vi "Pigeon2Configurator.vi"(6 "timeoutSeconds":dbl=0.05, 8 "error in":errorcluster, 10 "DeviceConfiguration":T2, 11 "DeviceReference":T1) -> (0 "error out":errorcluster)   [LabVIEW 2023]
uses:
  <vilib>/Rock Robotics/WPI/ThirdParty/Phoenix6/DeviceReference.ctl
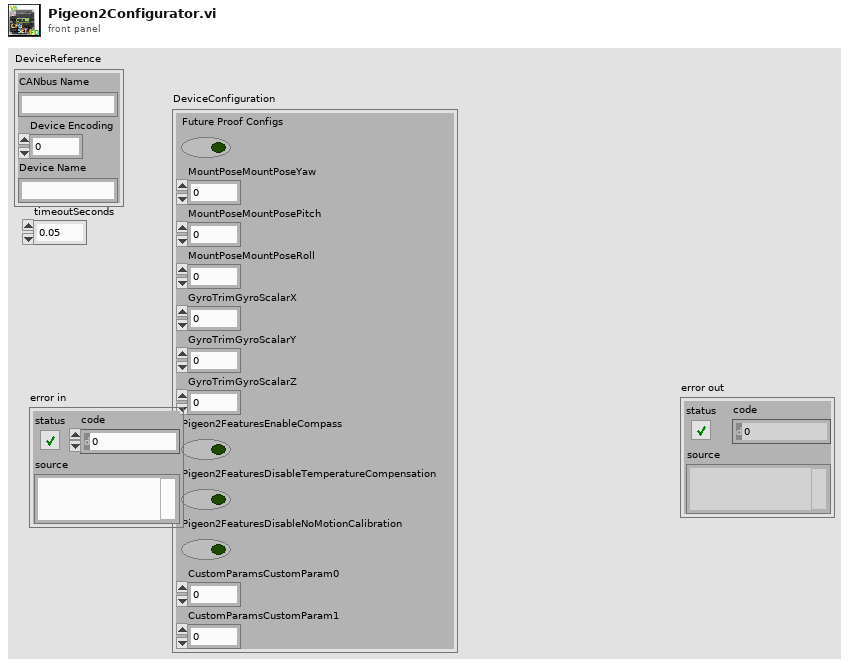
[diagram p1: front panel]
types:
  T1 = typedef "DeviceReference.ctl" = cluster{"CANbus Name":string, "Device Encoding":u32, "Device Name":string}
  T2 = cluster{"Future Proof Configs":bool, "MountPoseMountPoseYaw":dbl, "MountPoseMountPosePitch":dbl, "MountPoseMountPoseRoll":dbl, "GyroTrimGyroScalarX":dbl, "GyroTrimGyroScalarY":dbl, "GyroTrimGyroScalarZ":dbl, "Pigeon2FeaturesEnableCompass":bool, "Pigeon2FeaturesDisableTemperatureCompensation":bool, "Pigeon2FeaturesDisableNoMotionCalibration":bool, "CustomParamsCustomParam0":i16, "CustomParamsCustomParam1":i16}
  T3 = enum8{"<Null>", "I8", "I16", "I32", "I64", "U8", "U16", "U32", "U64", "SGL", "DBL", "EXT", "CSG", "CDB", "CXT", "0x0F", "0x10", "0x11", "0x12", "0x13", "0x14", "Enum U8", "Enum U16", "Enum U32", "Enum U64", "SGL PQ", "DBL PQ", "EXT PQ", "CSG PQ", "CDB PQ", "CXT PQ", "0x1F", "0x20", "Boolean", "0x22", "0x23", "0x24", "0x25", "0x26", "0x27", "0x28", "0x29", "0x2A", "0x2B", "0x2C", "0x2D", "0x2E", "0x2F", "String", "0x31", "Path", "Pict", "0x34", "0x35", "0x36", "DAQ", "0x38", "0x39", "0x3A", "0x3B", "0x3C", "0x3D", "0x3E", "0x3F", "Array", "0x41", "0x42", "0x43", "0x44", "0x45", "0x46", "0x47", "0x48", "0x49", "0x4A", "0x4B", "0x4C", "0x4D", "0x4E", "0x4F", "Cluster", "0x51", "0x52", "Variant", "Waveform", "0x55", "0x56", "0x57", "0x58", "0x59", "0x5A", "0x5B", "0x5C", "0x5D", "0x5E", "Fixed Point", "0x60", "0x61", "0x62", "0x63", "0x64", "0x65", "0x66", "0x67", "0x68", "0x69", "0x6A", "0x6B", "0x6C", "0x6D", "0x6E", "0x6F", "Refnum", "0x71", "0x72", "Set Collection", "Map Collection"}
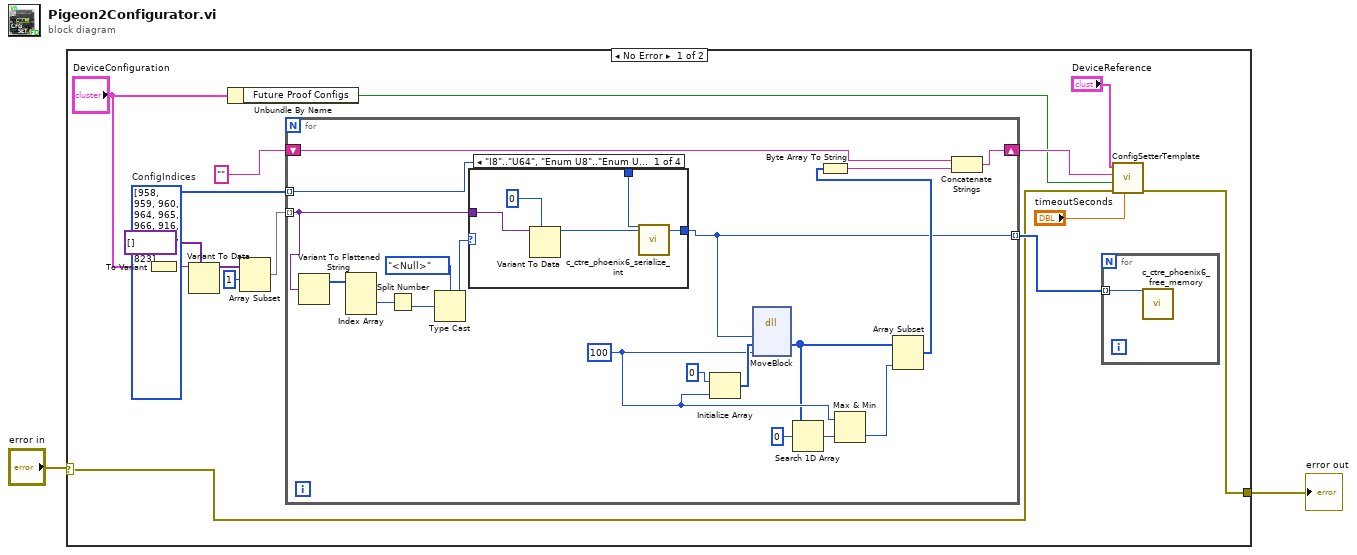
[diagram p0: block diagram]
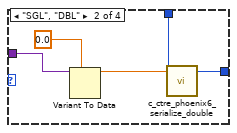
[diagram p2: hidden frame]
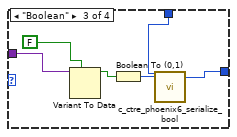
[diagram p3: hidden frame]
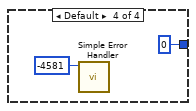
[diagram p4: hidden frame]
diagram:
  n1 = case shown="No Error" "error in" {
    selector: "error in" -> [w8 w56]
    tunnel: [w7 w56] -> w1
    frame No Error {
      w10 = i32[] [958, 959, 960, 964, 965, 966, 916, 951, 953, 822, 823]  # ConfigIndices
      n2 = To Variant(anything="DeviceConfiguration") -> (Variant=w6:variant)
      n3 = Variant To Data(type=variant[] [], Variant=w6) -> (data=w3:variant[])  [unwired: 1 in, 1 out]
      n4 = Unbundle By Name("DeviceConfiguration") -> ("Future Proof Configs"=w9:bool)
      n5 = Array Subset(array=w3, index=1) -> (w12:variant[])  [unwired: 1 in]
      n6 = for {
        tunnel: w12 -> [w19] mode=indexing
        shift-right: [w35] -> w16
        shift-left: "" -> [w36]
        tunnel: [w24] -> w11 mode=indexing
        tunnel: w10 -> [w25] mode=indexing
        w28 = i64 100 ("size")
        n7 = Variant To Flattened String(Variant=w19) -> (1:w22:i16[])  [unwired: 1 out]
        n8 = Index Array(array=w22) -> (element #2=w23:i16)  [unwired: 3 in, 2 out]
        n9 = Split Number(x=w23) -> (lo(x)=w20:u8)  [unwired: 1 out]
        n10 = Type Cast(type=T3."<Null>", x=w20) -> (*(type *) &x=w18:T3)
        n11 = case shown="\"I8\"..\"U64\", \"Enum U8\"..\"Enum U64\"" w18 {
          tunnel: w19 -> [w41 w46 w52 _]
          tunnel: w25 -> [w39 w43 w48 _]
          tunnel: [w37 w42 w47 u32 0 ("Numeric 4")] -> w24
          frame "I8".."U64", "Enum U8".."Enum U64" {
            n12 = Variant To Data(type=0, Variant=w41) -> (data=w38:i32)  [unwired: 1 in, 1 out]
            n13 = call <vilib>:"c_ctre_phoenix6_serialize_int.vi"("Numeric 2"=w39, "Numeric 3"=w38) -> ("Numeric 4"=w37:u32)  [unwired: 24 in, 1 out]
          }
          frame "SGL", "DBL" {
            n14 = Variant To Data(type=0.0, Variant=w46) -> (data=w44:dbl)  [unwired: 1 in, 1 out]
            n15 = call <vilib>:"c_ctre_phoenix6_serialize_double.vi"("Numeric 2"=w43, "Numeric 3"=w44) -> ("Numeric 4"=w42:u32)  [unwired: 24 in, 1 out]
          }
          frame "Boolean" {
            n16 = Variant To Data(type=FALSE, Variant=w52) -> (data=w50:bool)  [unwired: 1 in, 1 out]
            n17 = Boolean To (0,1)(Boolean=w50) -> (0, 1=w49:i16)
            n18 = call <vilib>:"c_ctre_phoenix6_serialize_bool.vi"("Numeric 2"=w48, "Numeric 3"=w49) -> ("Numeric 4"=w47:u32)  [unwired: 24 in, 1 out]
          }
          frame Default {
            n19 = call <vilib>:"Simple Error Handler.vi"("error code (no error:0)"=-4581) -> ()  [unwired: 4 in, 5 out]
          }
        }
        n20 = Initialize Array(u8 0 ("element"), w28) -> (w33:u8[])
        n21 = dll-call lib="LabVIEW" fn="MoveBlock"("ps"=w24, "pd"=w33, "size"=w28) -> ("pd"=w27:u8[])  [unwired: 6 in, 2 out]
        n22 = Search 1D Array(1D array=w27, element=u8 0) -> (index of element=w29:i32)  [unwired: 1 in]
        n23 = Max & Min(x=w28, y=w29) -> (min(x,y)=w26:i64)  [unwired: 1 out]
        n24 = Array Subset(array=w27, length=w26) -> (w31:u8[])  [unwired: 1 in]
        n25 = Byte Array To String(unsigned byte array=w31) -> (string=w34:string)
        n26 = Concatenate Strings(w36, w34) -> (w35:string)
      }
      n27 = for {
        tunnel: w11 -> [w55] mode=indexing
        n28 = call <vilib>:"c_ctre_phoenix6_free_memory.vi"("Numeric 3"=w55) -> ()  [unwired: 25 in, 2 out]
      }
      n29 = call <vilib>:"ConfigSetterTemplate.vi"("timeoutSeconds"="timeoutSeconds", "error in"=w8, "FutureProofConfigs"=w9, "Configs"=w16, "DeviceReference"="DeviceReference") -> ("error out"=w7:errorcluster)  [unwired: 6 in]
    }
    frame Error {
    }
  }
  "error out" <- w1
